vi "电流曲线2.vi"(5 "0安培电流保持时长":dbl=60.0, 6 "总持续时间3":dbl, 8 "总持续时间2":dbl, 9 "总持续时间1":dbl, 10 "时间分辨率":dbl, 11 "IR":dbl) -> (2 "最终电流值":dbl[](array[numeric]))   [LabVIEW 2012]
panel:
  out "输出电流值3":dbl[](array[numeric])
  out "稳态电流3":dbl
  out "输出电流值2":dbl[](array[numeric])
  out "稳态电流2":dbl
  out "输出电流值1":dbl[](array[numeric])
  out "稳态电流1":dbl
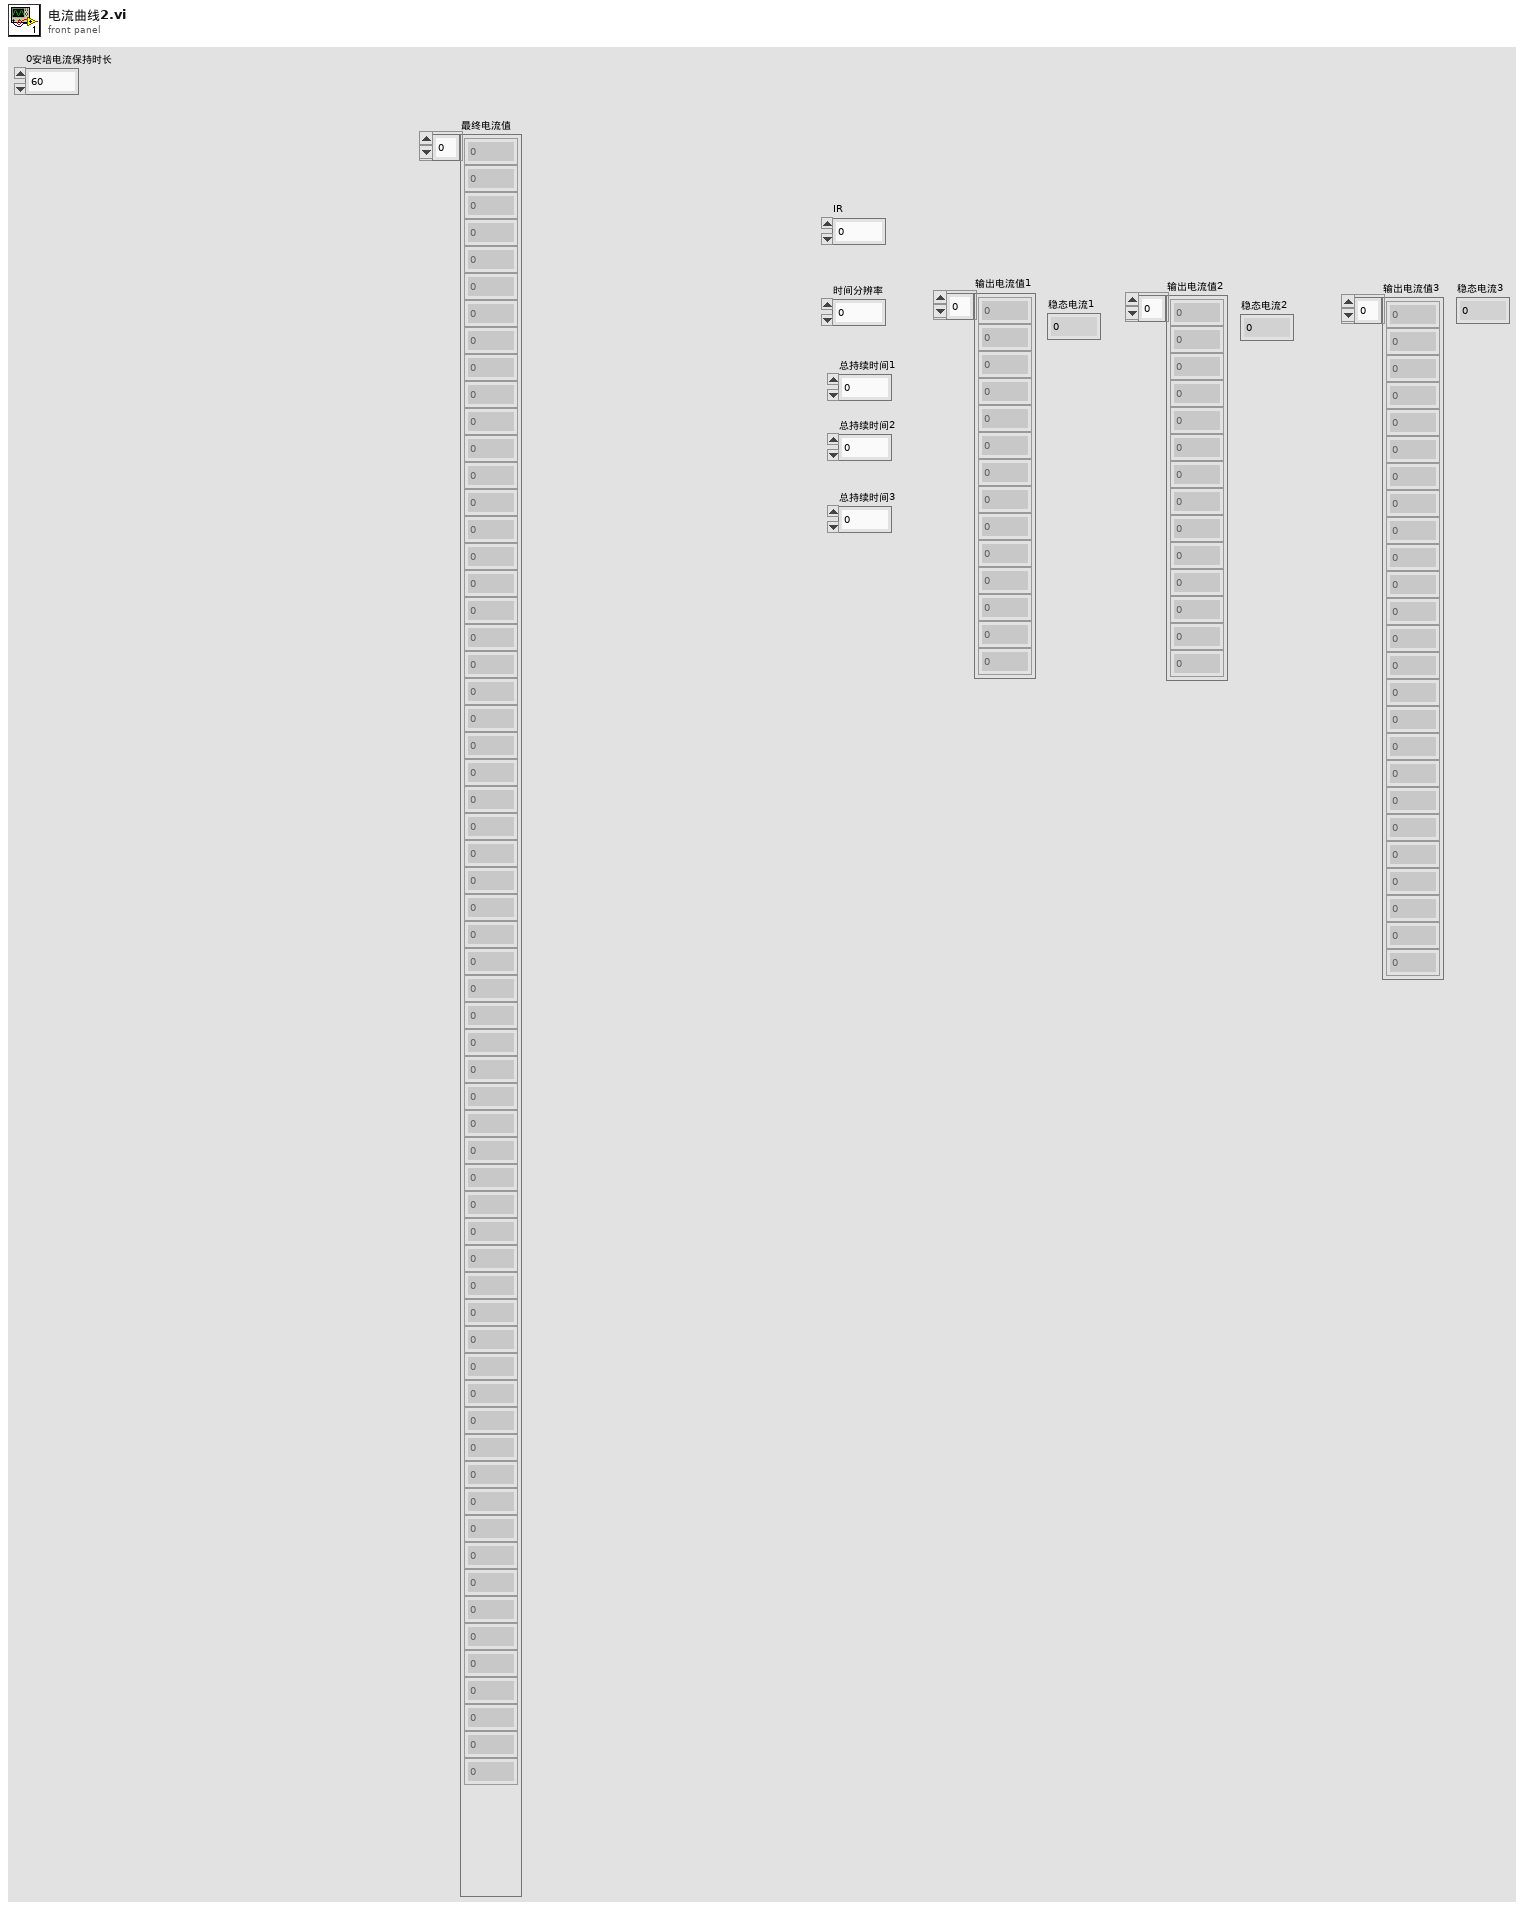
[diagram p1: front panel]
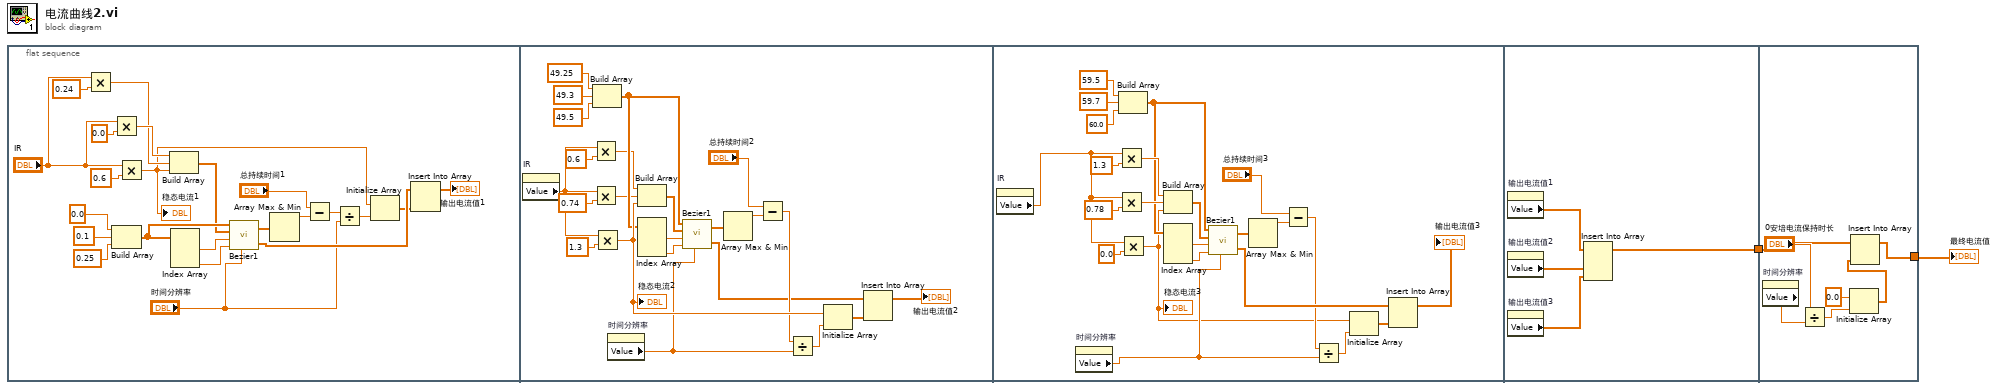
[diagram p0: block diagram]
diagram:
  n1 = flat-sequence {
    tunnel: [w72] -> w1
    tunnel: w1 -> [w77]
    tunnel: [w76] -> w2
    frame #0 {
      n2 = Multiply(x="IR", y=0.24) -> (x*y=w17:dbl)
      n3 = Multiply(x="IR", y=0.0) -> (x*y=w18:dbl)
      n4 = Build Array(0.0 ("元素"), 0.1 ("元素"), 0.25 ("元素")) -> (w16:dbl[])
      n5 = Multiply(x="IR", y=0.6) -> (x*y=w10:dbl)
      "稳态电流1" <- w10
      n6 = Build Array(w18, w17, w10) -> (w13:dbl[])
      n7 = Index Array(array=w16) -> (element #1=w15:dbl, element #3=w14:dbl)  [unwired: 3 in, 1 out]
      n8 = call "Bezier1.vi"("d"="时间分辨率", "y"=w14, "x"=w15, "Y"=w13, "X"=w16) -> ("查询的y"=w12:dbl[], "待查找值"=w9:dbl[])  [unwired: 1 in]
      n9 = Array Max & Min(array=w9) -> (max value=w8:dbl)  [unwired: 3 out]
      n10 = Subtract(x="总持续时间1", y=w8) -> (x-y=w6:dbl)
      n11 = Divide(x=w6, y="时间分辨率") -> (x/y=w4:dbl)
      n12 = Initialize Array(w10, w4) -> (w11:dbl[])
      n13 = Insert Into Array(array=w12, new element=w11) -> (→"输出电流值1":dbl[])  [unwired: 1 in]
    }
    frame #1 {
      n14 = property on="IR" class="DigNum (严格)"() -> ("Value"=w28:dbl)  [unwired: 2 in, 2 out]
      n15 = Multiply(x=w28, y=0.6) -> (x*y=w35:dbl)
      n16 = Multiply(x=w28, y=0.74) -> (x*y=w36:dbl)
      n17 = Build Array(49.25 ("元素"), 49.3 ("元素"), 49.5 ("元素")) -> (w37:dbl[])
      n18 = Multiply(x=w28, y=1.3) -> (x*y=w47:dbl)
      "稳态电流2" <- w47
      n19 = property on="时间分辨率" class="DigNum (严格)"() -> ("Value"=w45:dbl)  [unwired: 2 in, 2 out]
      n20 = Build Array(w35, w36, w47) -> (w40:dbl[])
      n21 = Index Array(array=w37) -> (element #1=w38:dbl, element #3=w39:dbl)  [unwired: 3 in, 1 out]
      n22 = call "Bezier1.vi"("d"=w45, "y"=w39, "x"=w38, "Y"=w40, "X"=w37) -> ("查询的y"=w42:dbl[], "待查找值"=w41:dbl[])  [unwired: 1 in]
      n23 = Array Max & Min(array=w41) -> (max value=w43:dbl)  [unwired: 3 out]
      n24 = Subtract(x="总持续时间2", y=w43) -> (x-y=w44:dbl)
      n25 = Divide(x=w44, y=w45) -> (x/y=w46:dbl)
      n26 = Initialize Array(w47, w46) -> (w48:dbl[])
      n27 = Insert Into Array(array=w42, new element=w48) -> (→"输出电流值2":dbl[])  [unwired: 1 in]
    }
    frame #2 {
      n28 = property on="IR" class="DigNum (严格)"() -> ("Value"=w70:dbl)  [unwired: 2 in, 2 out]
      n29 = property on="时间分辨率" class="DigNum (严格)"() -> ("Value"=w71:dbl)  [unwired: 2 in, 2 out]
      n30 = Multiply(x=w70, y=1.3) -> (x*y=w62:dbl)
      n31 = Multiply(x=w70, y=0.78) -> (x*y=w61:dbl)
      n32 = Build Array(59.5 ("元素"), 59.7 ("元素"), 60.0 ("元素")) -> (w60:dbl[])
      n33 = Multiply(x=w70, y=0.0) -> (x*y=w51:dbl)
      "稳态电流3" <- w51
      n34 = Build Array(w62, w61, w51) -> (w57:dbl[])
      n35 = Index Array(array=w60) -> (element #1=w59:dbl, element #3=w58:dbl)  [unwired: 3 in, 1 out]
      n36 = call "Bezier1.vi"("d"=w71, "y"=w58, "x"=w59, "Y"=w57, "X"=w60) -> ("查询的y"=w55:dbl[], "待查找值"=w56:dbl[])  [unwired: 1 in]
      n37 = Array Max & Min(array=w56) -> (max value=w54:dbl)  [unwired: 3 out]
      n38 = Subtract(x="总持续时间3", y=w54) -> (x-y=w53:dbl)
      n39 = Divide(x=w53, y=w71) -> (x/y=w52:dbl)
      n40 = Initialize Array(w51, w52) -> (w50:dbl[])
      n41 = Insert Into Array(array=w55, new element=w50) -> (→"输出电流值3":dbl[])  [unwired: 1 in]
    }
    frame #3 {
      n42 = property on="输出电流值1" class="Arr (严格)"() -> ("Value"=w73:dbl[])  [unwired: 2 in, 2 out]
      n43 = property on="输出电流值2" class="Arr (严格)"() -> ("Value"=w74:dbl[])  [unwired: 2 in, 2 out]
      n44 = property on="输出电流值3" class="Arr (严格)"() -> ("Value"=w75:dbl[])  [unwired: 2 in, 2 out]
      n45 = Insert Into Array(array=w73, new element #1=w74, new element #2=w75) -> (w72:dbl[])  [unwired: 1 in]
    }
    frame #4 {
      n46 = property on="时间分辨率" class="DigNum (严格)"() -> ("Value"=w82:dbl)  [unwired: 2 in, 2 out]
      n47 = Divide(x="0安培电流保持时长", y=w82) -> (x/y=w80:dbl)
      n48 = Initialize Array(0.0 ("元素"), w80) -> (w78:dbl[])
      n49 = Insert Into Array(array=w77, new element=w78) -> (w76:dbl[])  [unwired: 1 in]
    }
  }
  "最终电流值" <- w2
